vi "zmq_send_multi.vi"(3 "error in":errorcluster, 4 "parts":string[](array[string]), 5 "socket in":refnum<class "Socket.lvclass">) -> (0 "error out":errorcluster, 2 "socket out":refnum<class "Socket.lvclass">)   [LabVIEW 2025, in "ZeroMQ.lvlib" / "Socket.lvclass"]
doc: "Sends a multi-component message corresponding to the elements of <b>parts</b> through the socket."
uses:
  Socket.lvclass
  Socket.lvclass/Socket.ctl
  ZeroMQ.lvlib
panel:
  # "ØMQ"
  # "labview"
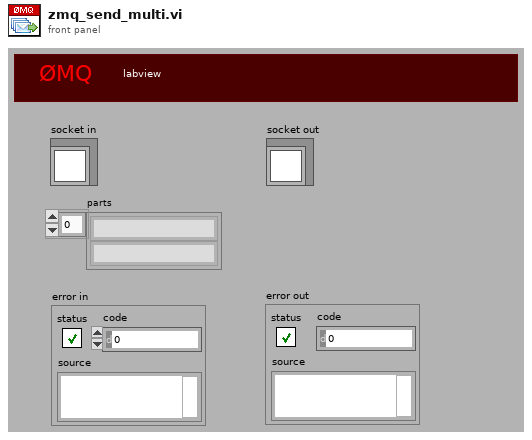
[diagram p1: front panel]
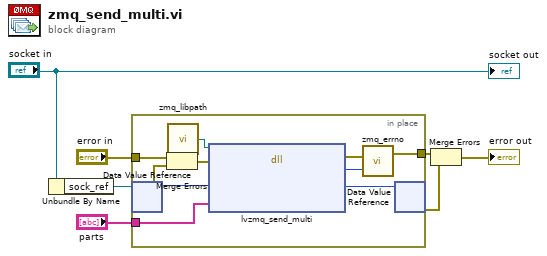
[diagram p0: block diagram]
diagram:
  n1 = Unbundle By Name("socket in") -> ("sock_ref"=w3:refnum<data-value>)
  n2 = in-place {
    in-place-border: "parts" -> [w15]
    in-place-border: "error in" -> [w14]
    in-place-border: [w13] -> w5
    n3 = in-place-dvr #1(w3) -> (w12:u64, w8:errorcluster)
    n4 = Merge Errors(w14, w8) -> (w9:errorcluster)
    n5 = call "zmq_libpath.vi"() -> ("path"=w10:path)
    n6 = dll-call lib="?" fn="lvzmq_send_multi" ("zmq_labview.dll:lvzmq_socket")(path in=w10, error in=w9, "sock_obj"=w12, "data"=w15) -> (error out=w17:errorcluster, "return type"=w16:i32, "sock_obj"=w11:u64)  [unwired: 2 in, 1 out]
    n7 = call "zmq_errno.vi"("retval"=w16, "error in"=w17) -> ("error out"=w13:errorcluster)  [unwired: 1 out]
    n8 = in-place-dvr #1(w11) -> (w1:errorcluster)  [unwired: 1 out]
  }
  n9 = Merge Errors(w5, w1) -> (→"error out":errorcluster)
  "socket out" <- "socket in"
